vi "sample-rate-trigger.vi"(0 "last-event-mS in":u32=1 min=1 max=4, 2 "Sample Rate (Hz)":dbl=1.0 min=0.0001 max=4.0 format="%#_4g", 3 "mS modifyer":i32=1) -> (5 "Delay Time":u32, 6 "triggered?":bool, 7 "last-event-mS out":u32=1 min=1 max=4, 9 "Elapsed Time mS":u32=1 min=1 max=4)   [LabVIEW 2020]
panel:
  # "This to account for loop time"
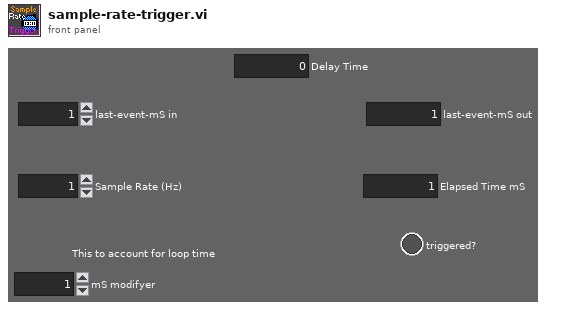
[diagram p1: front panel]
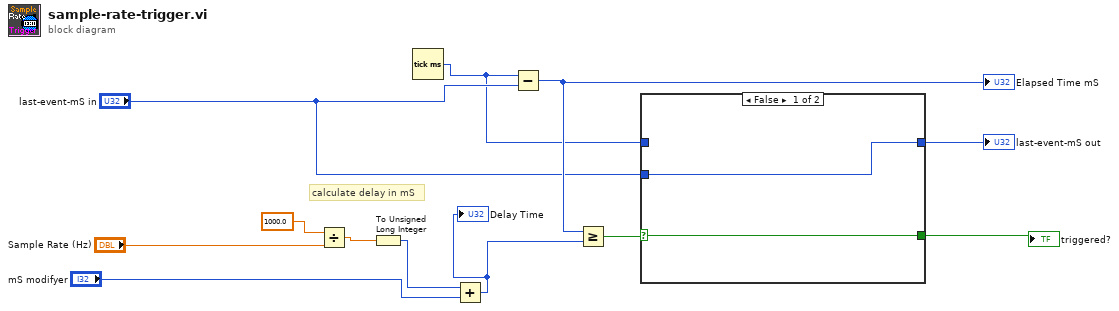
[diagram p0: block diagram]
diagram:
  # "calculate delay in mS"
  n1 = Divide(x=1000.0 ("milliseconds to wait"), y="Sample Rate (Hz)") -> (x/y=w12:dbl)
  n2 = To Unsigned Long Integer(number=w12) -> (unsigned 32bit integer=w3:u32)
  n3 = Tick Count (ms)() -> (millisecond timer value=w5:u32)
  n4 = Add(x=w3, y="mS modifyer") -> (x+y=w1:u32)
  "Delay Time" <- w1
  n5 = Subtract(x=w5, y="last-event-mS in") -> (x-y=w9:u32)
  "Elapsed Time mS" <- w9
  n6 = Greater Or Equal?(x=w9, y=w1) -> (x >= y?=w8:bool)
  n7 = case shown="False" w8 {
    selector: w8 -> [w13 w15]
    tunnel: [w14 w16] -> w7
    tunnel: "last-event-mS in" -> [w14 _]
    tunnel: w5 -> [_ w16]
    tunnel: [w13 w15] -> w4
    frame False {
    }
    frame True {
    }
  }
  "last-event-mS out" <- w7
  "triggered?" <- w4
